vi "3DAccel.vi"() -> ()   [LabVIEW 2019]
uses:
  <vilib>/MakerHub/LINX/Public/Sensors/Accelerometer/MPU60X0/DeviceAddresses.ctl
  <vilib>/MakerHub/LINX/Public/Utilities/Open Serial.vi
  <vilib>/picture/3D Picture Control/Object/Create Object (drawable).vi
  <vilib>/MakerHub/LINX/LMH-LINX.lvlib
  <vilib>/MakerHub/LINX/Public/Sensors/Accelerometer/MPU60X0/MPU60X0.lvlib
  <vilib>/picture/3D Picture Control/NI_3D Picture Control.lvlib
panel:
  in  "Angle":sgl
  out "3D Picture":refnum<vi>(3d-picture)
  in  "stop":bool
  out "Acceleration Data (g)":T1
  in  "Serial Port":refnum<visa-resource-name>="N/A"
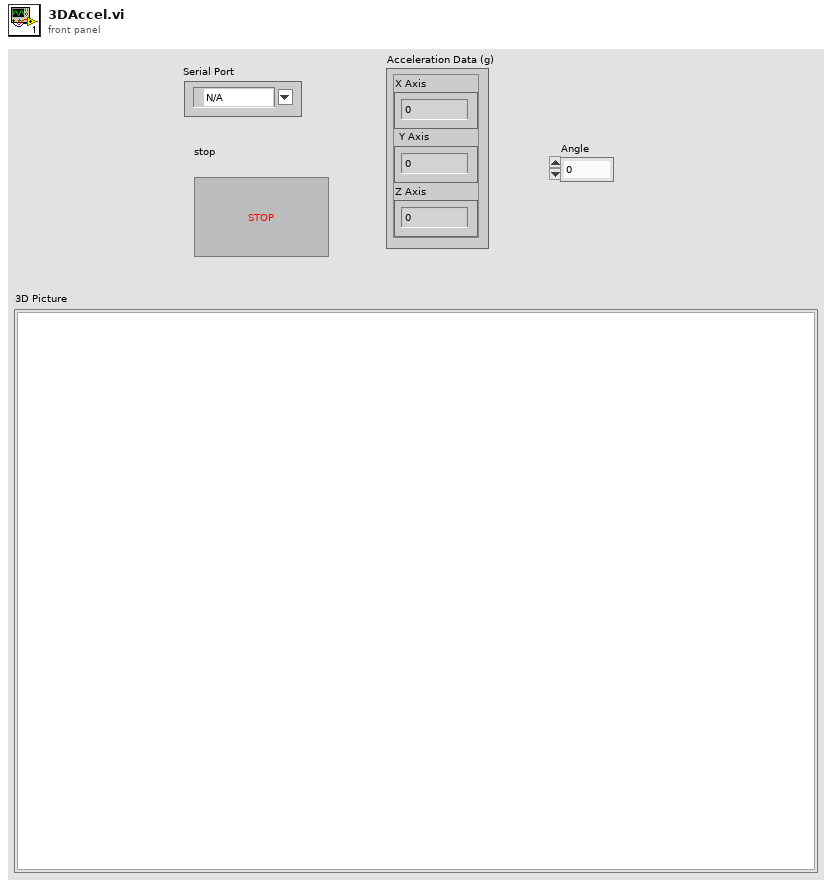
[diagram p1: front panel]
types:
  T1 = cluster{"X Axis":i16, "Y Axis":i16, "Z Axis":i16}
  T2 = typedef "LMH-LINX.lvlib/MPU60X0.lvlib/DeviceAddresses.ctl" = enum16{"0x68", "0x69"}
  T3 = typedef "LMH-LINX.lvlib/LINX Ref.ctl" = cluster{"IO":T4, "Interface":T5, "LINX Device Config":T6}
  T4 = typedef "LMH-LINX.lvlib/Platform.ctl" = enum16{"Remote", "Local"}
  T5 = typedef "LMH-LINX.lvlib/Interface.ctl" = enum16{"Serial", "TCP"}
  T6 = typedef "LMH-LINX.lvlib/Device.lvlib/LINX Device Config.ctl" = cluster{"Interface":T5, "COM Port":refnum<visa-resource-name>, "TCP Configuration":T7, "Device Family":u8, "Device ID":u8, "Device Name":string, "TCP Ref":refnum<k5>, "Channels":T8}
  T7 = typedef "LMH-LINX.lvlib/Device.lvlib/TCP Config.ctl" = cluster{"IP Address":string, "Port":u16}
  T8 = typedef "LMH-LINX.lvlib/Channels.ctl" = cluster{"DI":u8[], "DO":u8[], "AI":u8[], "AO":u8[], "PWM":u8[], "QE":u8[], "UART":u8[], "I2C 2":u8[], "SPI":u8[], "CAN":u8[], "Servo":u8[], "AI Ref (V)":dbl, "AI Resolution (Bits)":u8, "AO Ref (V)":dbl, "AO Resolution (Bits)":u8}
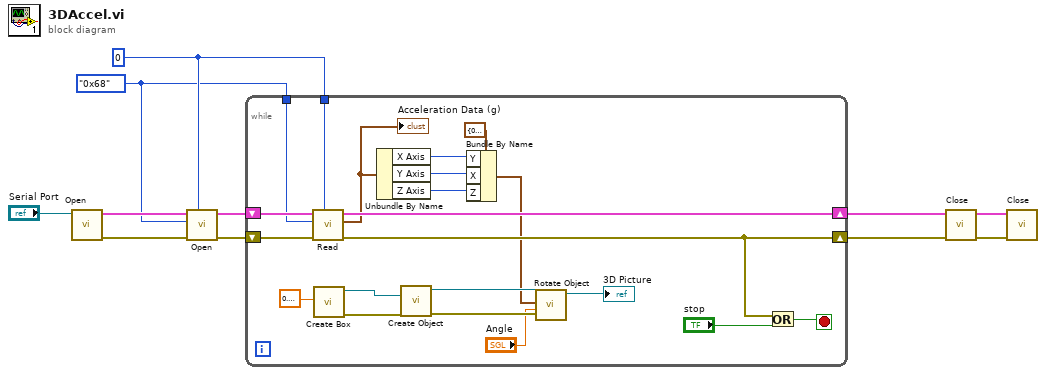
[diagram p0: block diagram]
diagram:
  w2 = u8 0 ("I2C Channel")
  w1 = DeviceAddresses."0x68" ("I2C Slave Address")
  n1 = call-poly <vilib>:"Open.vi"("Serial Port"="Serial Port") -> ("Error Out"=w10:errorcluster, "LINX Resource"=w11:T3)  [unwired: 8 in, 1 out]
  n2 = call <vilib>:"Open.vi"("I2C Channel"=w2, "Error In"=w10, "I2C Slave Address"=w1, "LINX Resource"=w11) -> ("Error Out"=w8:errorcluster, "LINX Resource"=w9:T3)  [unwired: 6 in]
  n3 = while {
    shift-right: [w30] -> w7
    shift-left: w9 -> [w32]
    shift-right: [w27] -> w6
    shift-left: w8 -> [w31]
    tunnel: w2 -> [w29]
    tunnel: w1 -> [w28]
    stop <- w25 stop-if-true
    n4 = call <vilib>:"Read.vi"("I2C Channel"=w29, "Error In"=w31, "I2C Slave Address"=w28, "LINX Resource"=w32) -> ("Error Out"=w27:errorcluster, "Acceleration Data (g)"=w18:T1, "LINX Resource"=w30:T3)  [unwired: 3 in, 2 out]
    "Acceleration Data (g)" <- w18
    n5 = call <vilib>:"Create Box.vi"("Length Y"=sgl 0.2) -> ("error out"=w21:errorcluster, "New Box Refnum"=w20:refnum<vi>)  [unwired: 9 in]
    n6 = Unbundle By Name(w18) -> ("X Axis"=w16:i16, "Y Axis"=w15:i16, "Z Axis"=w14:i16)
    n7 = call-poly <vilib>:"Create Object.vi"("error in (no error)"=w21, "Geometry"=w20) -> ("error out"=w23:errorcluster, "Scene:New Object"=w22:refnum<vi>)  [unwired: 8 in]
    n8 = Bundle By Name(cluster=cluster{"X":sgl, "Y":sgl, "Z":sgl} {"X"=0.0, "Y"=0.0, "Z"=0.0} ("Axis"), "Y"=w16, "X"=w15, "Z"=w14) -> (w13:cluster{"X":sgl, "Y":sgl, "Z":sgl})
    n9 = call <vilib>:"Rotate Object.vi"("error in (no error)"=w23, "Angle"="Angle", "Axis"=w13, "Scene.Object In"=w22) -> ("Scene.Object Out"=→"3D Picture":refnum<vi>)  [unwired: 6 in, 1 out]
    n10 = Or(x=w27, y="stop") -> (x .or. y?=w25:bool)
  }
  n11 = call <vilib>:"Close.vi"("Error In"=w6, "LINX Resource"=w7) -> ("Error Out"=w4:errorcluster, "LINX Resource"=w5:T3)  [unwired: 8 in]
  n12 = call <vilib>:"Close.vi"("Error In"=w4, "LINX Resource"=w5) -> ()  [unwired: 9 in, 1 out]
